vi "gfd.vi"() -> ()   [LabVIEW 2011]
panel:
  out "x+y":dbl[](array[numeric])
  in  "Array 2":dbl[](array[numeric])
  in  "Array":dbl[](array[numeric])
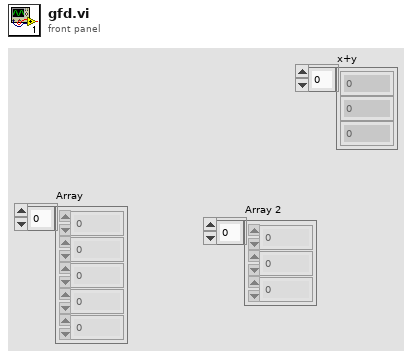
[diagram p1: front panel]
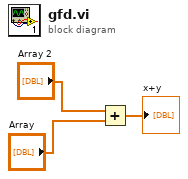
[diagram p0: block diagram]
diagram:
  n1 = Add(x="Array 2", y="Array") -> (x+y=→"x+y":dbl[])
